vi "Joystick Layout.vi"() -> ()   [LabVIEW 2015]
uses:
  <vilib>/Rock Robotics/WPI/Utilities/WPI_GetSetVariantRefNum.vi
panel:
  in  "Joystick Name":string
  out "Buttons":T1
  out "Axis":T2
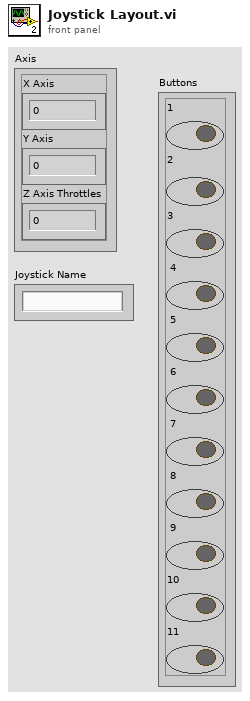
[diagram p1: front panel]
types:
  T1 = cluster{"1":bool, "2":bool, "3":bool, " 4":bool, " 5":bool, " 6":bool, " 7":bool, " 8":bool, " 9":bool, "10":bool, "11":bool}
  T2 = cluster{"X Axis":dbl, "Y Axis":dbl, "Z Axis Throttles":dbl}
  T3 = typedef "WPI_JoystickDevRef.ctl" = cluster{"Device":T4}
  T4 = typedef "WPI_JoystickDeviceEnum.ctl" = enum16{"USB 0", "USB 1", "USB 2", "USB 3", "USB 4", "USB 5"}
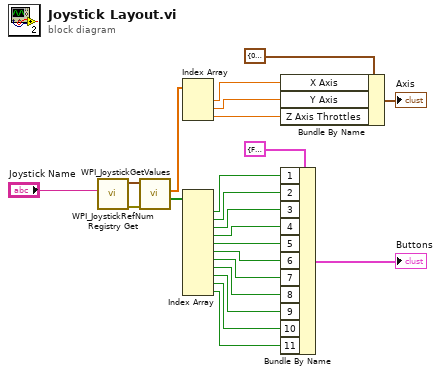
[diagram p0: block diagram]
diagram:
  n1 = call <vilib>:"WPI_JoystickRefNum Registry Get.vi"("refnum name"="Joystick Name") -> ("error out"=w23:errorcluster, "JoystickDevRef"=w22:T3)  [unwired: 9 in]
  n2 = call <vilib>:"WPI_JoystickGetValues.vi"("error in (no error)"=w23, "JoystickDevRef"=w22) -> ("Buttons"=w20:bool[], "Axes"=w6:dbl[])  [unwired: 5 in, 3 out]
  n3 = Index Array(array=w6) -> (element #1=w4:dbl, element #2=w3:dbl, element #3=w2:dbl)  [unwired: 3 in]
  n4 = Index Array(array=w20) -> (element #1=w17:bool, element #2=w16:bool, element #3=w15:bool, element #4=w14:bool, element #5=w13:bool, element #6=w12:bool, element #7=w11:bool, element #8=w10:bool, element #9=w9:bool, element #10=w8:bool, element #11=w7:bool)  [unwired: 11 in]
  n5 = Bundle By Name(cluster=T2 {"X Axis"=0.0, "Y Axis"=0.0, "Z Axis Throttles"=0.0} ("Axis"), "X Axis"=w4, "Y Axis"=w3, "Z Axis Throttles"=w2) -> (→"Axis":T2)
  n6 = Bundle By Name(cluster=T1 {"1"=FALSE, "2"=FALSE, "3"=FALSE, " 4"=FALSE, " 5"=FALSE, " 6"=FALSE, " 7"=FALSE, " 8"=FALSE, " 9"=FALSE, "10"=FALSE, "11"=FALSE} ("Buttons"), "1"=w17, "2"=w16, "3"=w15, "4"=w14, "5"=w13, "6"=w12, "7"=w11, "8"=w10, "9"=w9, "10"=w8, "11"=w7) -> (→"Buttons":T1)
